vi "Write Section Cluster__ogtk.vi"(5 "float number format (optional)":string, 7 "section (optional)":string, 8 "error in (no error)":errorcluster, 10 "Section Formatted Cluster":variant, 11 "refnum":T1) -> (0 "error out":errorcluster, 3 "dup refnum":T1)   [LabVIEW 2011]
doc: "Writes key-value pairs to a section of the configuration data identified by refnum, which correspond to the named items and thier values within the \"Section Formatted Cluster\" input. If \"key\" input is not specified, the name of the cluster within the \"Section Formatted Cluster\" input is used as the key.\n\nFor example an section cluster named \"MyCluster1\" contains two elements named \"MyNumeric\" and \"MyBoolean\". This would correspond to an INI write of the following data:\n\n[MyCluster1]\nMyNumeric=1.024\nMyBoolean=TRUE\n\nNote: Special characters in section and key names will be escape-coded. These include the following: \\00-\\1F (non-printable chars); \"[\", \"]\", and \"=\" (INI syntax elements); \\FE (\"þ\") and \\FF (\"ÿ\") (legacy bracket encoding); Additionally, the escape character, \"\\\", will be escaped as \"\\\\\"."
uses:
  <vilib>/Utility/config.llb/Config Data RefNum.ctl
  <vilib>/Utility/config.llb/NI_LVConfig.lvlib
panel:
  # "Write Variant Section Cluster.vi\n\nWrites an INI section cluster (variant) to INI file. \n\nPlease visit http://www.OpenG.org to learn about the\nOpen Source LabVIEW software movement.\n\nNOTICE -- YOU MUST LEAVE THIS NOTICE IN PLACE.  PER THE TERMS OF THE LICENSE BELOW, YOU MAY SUBLICENSE THIS SOFTWARE \nIN ANY WAY THAT DOES NOT CONFLICT WITH THIS LICENSE.\n\n### BSD License (http://www.opensource.org/licenses/bsd-license.php) Begin ###\n \nCopyright (c) 2002-2006, Jim Kring <jim@jimkring.com>\n\nAll rights reserved.\n\nRedistribution and use in source and binary forms, with or without modification, are permitted provided that the following conditions are met:\n\n    * Redistributions of source code must retain the above copyright notice, this list of conditions and the following disclaimer.\n    * Redistributions in binary form must reproduce the above copyright notice, this list of conditions and the following disclaimer in the \n       documentation and/or other materials provided with the distribution.\n    * Neither the name of SciWare, James Kring, Inc., nor the names of its contributors may be used to endorse or promote products derived \n       from this software without specific prior written permission.\n\nTHIS SOFTWARE IS PROVIDED BY THE COPYRIGHT HOLDERS AND CONTRIBUTORS \"AS IS\" AND ANY EXPRESS OR IMPLIED WARRANTIES, \nINCLUDING, BUT NOT LIMITED TO, THE IMPLIED WARRANTIES OF MERCHANTABILITY AND FITNESS FOR A PARTICULAR PURPOSE ARE \nDISCLAIMED. IN NO EVENT SHALL THE COPYRIGHT OWNER OR CONTRIBUTORS BE LIABLE FOR ANY DIRECT, INDIRECT, INCIDENTAL,\n SPECIAL, EXEMPLARY, OR CONSEQUENTIAL DAMAGES (INCLUDING, BUT NOT LIMITED TO, PROCUREMENT OF SUBSTITUTE GOODS OR \nSERVICES; LOSS OF USE, DATA, OR PROFITS; OR BUSINESS INTERRUPTION) HOWEVER CAUSED AND ON ANY THEORY OF LIABILITY, \nWHETHER IN CONTRACT, STRICT LIABILITY, OR TORT (INCLUDING NEGLIGENCE OR OTHERWISE) ARISING IN ANY WAY OUT OF THE USE \nOF THIS SOFTWARE, EVEN IF ADVISED OF THE POSSIBILITY OF SUCH DAMAGE.\n\n### BSD License End ###"
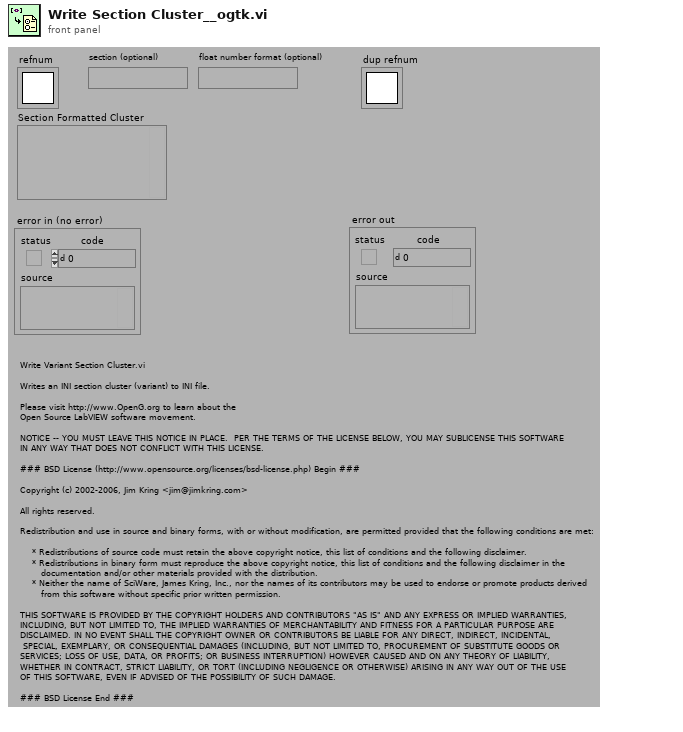
[diagram p1: front panel]
types:
  T1 = typedef "NI_LVConfig.lvlib/Config Data RefNum.ctl" = refnum<k1>
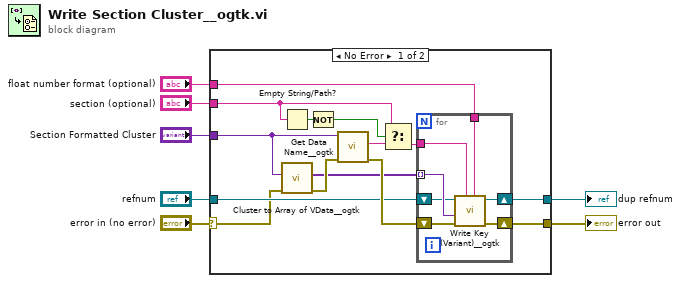
[diagram p0: block diagram]
diagram:
  n1 = case shown="No Error" "error in (no error)" {
    selector: "error in (no error)" -> [w8 w30]
    tunnel: [w19 w30] -> w7
    tunnel: [w18 w29] -> w6
    tunnel: "refnum" -> [w17 w29]
    tunnel: "section (optional)" -> [w14 _]
    tunnel: "Section Formatted Cluster" -> [w10 _]
    tunnel: "float number format (optional)" -> [w9 _]
    frame No Error {
      n2 = Empty String/Path?(string/path=w14) -> (empty?=w15:bool)
      n3 = call <userlib>:"Cluster to Array of VData__ogtk.vi"("error in (no error)"=w8, "Cluster"=w10) -> ("error out"=w20:errorcluster, "Array of VData"=w16:variant[])  [unwired: 8 in]
      n4 = Not(x=w15) -> (.not. x?=w13:bool)
      n5 = call <userlib>:"Get Data Name__ogtk.vi"("error in (no error)"=w20, "Data"=w10) -> ("error out"=w21:errorcluster, "Data Name"=w12:string)  [unwired: 7 in, 1 out]
      n6 = Select(t=w14, s=w13, f=w12) -> (s? t:f=w11:string)
      n7 = for {
        tunnel: w16 -> [w28] mode=indexing
        shift-right: [w24] -> w18
        shift-left: w17 -> [w27]
        shift-right: [w25] -> w19
        shift-left: w21 -> [w26]
        tunnel: w11 -> [w23]
        tunnel: w9 -> [w22]
        n8 = call <userlib>:"Write Key (Variant)__ogtk.vi"("float number format"=w22, "section"=w23, "error in (no error)"=w26, "key-value"=w28, "refnum"=w27) -> ("error out"=w25:errorcluster, "refnum out"=w24:T1)  [unwired: 5 in]
      }
    }
    frame Error {
    }
  }
  "error out" <- w7
  "dup refnum" <- w6
